vi "Camera_init.vi"(8 "error in":errorcluster, 11 "input cluster":T1={"L16 Linear Actuator"="", "XE 1000 Pump"="", "Camera1"="", "Camera2"="", "Img_Capt"=FALSE, "Actuator"=FALSE, "Pump"=FALSE, "Cam 1"=FALSE, "Cam 2"=FALSE, "Empty_Refill"=FALSE, "Crop"=FALSE, "Light intensity"=100, "Exposure Time"=1000.0, "Sample Name"="Test Sample", "Operator"="MRJ", "Calibration 1"=path "C:/Users/au540322/Desktop/IHS_Project/images/Debris/Debris_0/Debris_0_2019_06_01-23-32-49-686.PNG", "Calibration 2"=path "C:/Users/au540322/Desktop/IHS_Project/images/Debris/Debris_0/Debris_0_2019_06_01-23-32-49-686.PNG", "Framerate"=1, "Timeout Sample"=0, "Collection date"="MRJ", "Sample size threshold"=1, "Empty start"=1, "Command"="MRJ", "Station"="", "Species Name"="", "Other Notes"="", "Aperture"=enum."Item 0", "Image Process Queue Size"=500, "Image Save Queue Size"=500, "Overload threshold"=500, "Max Framerate"=100, "Rectangle 1"={"Left"=0, "Top"=0, "Right"=0, "Bottom"=0, "Rotation"=0.0}, "Rectangle 2"={"Left"=0, "Top"=0, "Right"=0, "Bottom"=0, "Rotation"=0.0}, "Detection Region %"=0.0, "Detect 1"=path "C:/Users/au540322/Desktop/IHS_Project/images/Debris/Debris_0/Debris_0_2019_06_01-23-32-49-686.PNG", "Detect 2"=path "C:/Users/au540322/Desktop/IHS_Project/images/Debris/Debris_0/Debris_0_2019_06_01-23-32-49-686.PNG", "Max large object threshold"=0, "Open(T)/Close(F)"=FALSE, "Img_Capt Begin"=FALSE, "Dispense Speed"=100, "Flush Size"=100, "Location"="Station", "Latitude"="Station", "Longitude"="Station", "Determiner"="Station", "Sex"="Station", "Camera1_Img"=refnum, "Camera2_Img"=refnum, "Img1_Orig_Disp"=refnum, "Img2_Orig_Disp"=refnum, "Img1_Orig_RGB"=refnum, "Img2_Orig_RGB"=refnum, "Blue_Plane_Extract"=refnum, "Subtracted_Plane"=refnum, "Img1_Binary"=refnum, "Img2_Binary"=refnum, "Crop_Mask"=refnum, "Img1_Save"=refnum, "Img2_Save"=refnum, "Img1_Cali_Full"=refnum, "Img2_Cali_Full"=refnum, "Img1_Cali_Detect"=refnum, "Img2_Cali_Detect"=refnum, "Cam 1 queue"=refnum, "Cam 2 queue"=refnum, "Cam 1 - save queue"=refnum, "Cam 2 - save queue"=refnum, "Overlay_Ring"=0, "SystemVersion"=0, "System Serial"="", "Legacy Cam Attributes"=FALSE, "Camera Orientation 1"="", "Camera Orientation 2"="", "Pixel to mm 1"=0.0, "Pixel to mm 2"=0.0} {"SystemVersion" items=["Standard", "XL"]; "Overlay_Ring" items=["Session Data", "Extended Setup", "Buffer", "Camera", "Dispenser", "Stats", "Connections"]; "Flush Size" min=1; "Dispense Speed" min=1; "Rectangle 2"."Rotation" format="%.2f"; "Rectangle 2"."Left" scale=0.0..1024.0; "Rectangle 2"."Right" scale=0.0..1024.0; "Rectangle 1"."Rotation" format="%.2f"; "Rectangle 1"."Left" scale=0.0..1024.0; "Rectangle 1"."Right" scale=0.0..1024.0; "Max Framerate" min=1; "Overload threshold" min=1; "Image Save Queue Size" min=1; "Image Process Queue Size" min=1; "Empty start" min=1; "Sample size threshold" min=1; "Framerate" min=1; "Light intensity" scale=0.0..100.0}) -> (0 "Cam2 Status":bool, 1 "Cam1 Status":bool, 2 "Camera2":T2, 3 "Camera1":T2)   [LabVIEW 2022 SP3]
uses:
  <vilib>/userdefined/High Color/IMAQdx.ctl
  controls/Data.ctl
  <vilib>/vision/Image Controls.llb/IMAQ Image.ctl
  <vilib>/vision/driver/IMAQdx.llb/IMAQdx Camera Control Mode.ctl
  5e997588-f8a4-47c3-81e2-b2b6234dc64e.vi
  <vilib>/vision/driver/NI_Vision_Acquisition_Software.lvlib
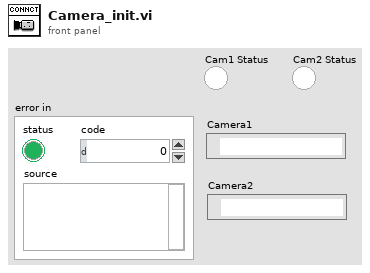
[diagram p1: front panel]
types:
  T1 = typedef "Data.ctl" = cluster{"L16 Linear Actuator":refnum<visa-resource-name>, "XE 1000 Pump":refnum<visa-resource-name>, "Camera1":T2, "Camera2":T2, "Img_Capt":bool, "Actuator":bool, "Pump":bool, "Cam 1":bool, "Cam 2":bool, "Empty_Refill":bool, "Crop":bool, "Light intensity":i32, "Exposure Time":dbl, "Sample Name":string, "Operator":string, "Calibration 1":path, "Calibration 2":path, "Framerate":i32, "Timeout Sample":i32, "Collection date":string, "Sample size threshold":i32, "Empty start":u32, "Command":string, "Station":string, "Species Name":string, "Other Notes":string, "Aperture":enum32{"Item 0", "Item 1", "Item 2", "Item 3"}, "Image Process Queue Size":i32, "Image Save Queue Size":i32, "Overload threshold":i32, "Max Framerate":i32, "Rectangle 1":T3, "Rectangle 2":T3, "Detection Region %":dbl, "Detect 1":path, "Detect 2":path, "Max large object threshold":i32, "Open(T)/Close(F)":bool, "Img_Capt Begin":bool, "Dispense Speed":i32, "Flush Size":i32, "Location":string, "Latitude":string, "Longitude":string, "Determiner":string, "Sex":string, "Camera1_Img":T4, "Camera2_Img":T4, "Img1_Orig_Disp":T4, "Img2_Orig_Disp":T4, "Img1_Orig_RGB":T4, "Img2_Orig_RGB":T4, "Blue_Plane_Extract":T4, "Subtracted_Plane":T4, "Img1_Binary":T4, "Img2_Binary":T4, "Crop_Mask":T4, "Img1_Save":T4, "Img2_Save":T4, "Img1_Cali_Full":T4, "Img2_Cali_Full":T4, "Img1_Cali_Detect":T4, "Img2_Cali_Detect":T4, "Cam 1 queue":refnum<queue>, "Cam 2 queue":refnum<queue>, "Cam 1 - save queue":refnum<queue>, "Cam 2 - save queue":refnum<queue>, "Overlay_Ring":u16, "SystemVersion":u16, "System Serial":string, "Legacy Cam Attributes":bool, "Camera Orientation 1":string, "Camera Orientation 2":string, "Pixel to mm 1":dbl, "Pixel to mm 2":dbl}
  T2 = typedef "IMAQdx.ctl" = refnum<k21>
  T3 = typedef "IMAQ Rectangle" = cluster{"Left":i32, "Top":i32, "Right":i32, "Bottom":i32, "Rotation":dbl}
  T4 = typedef "IMAQ Image.ctl" = refnum<image>
  T5 = typedef "CAM_ID.ctl" = cluster{"CAM_ID1":i32, "CAM_ID2":i32}
  T6 = typedef "NI_Vision_Acquisition_Software.lvlib/IMAQdx Camera Control Mode.ctl" = enum32{"Controller", "Listener"}
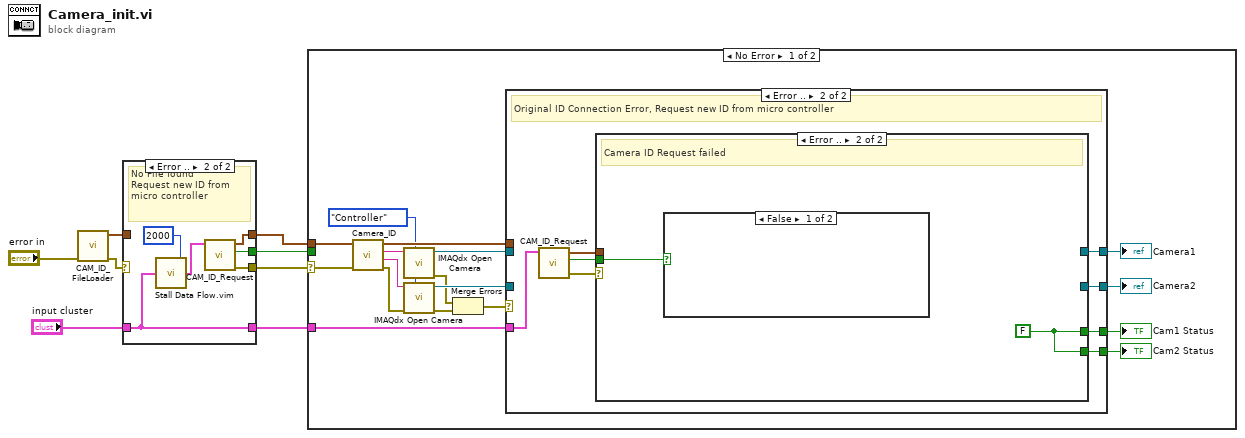
[diagram p0: block diagram]
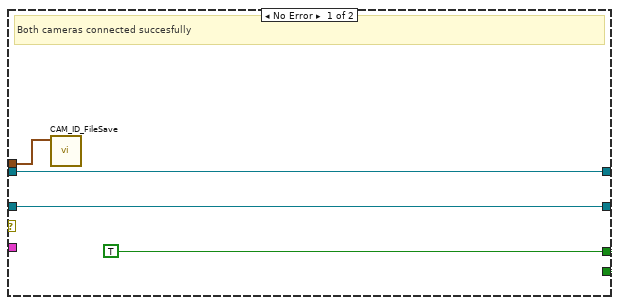
[diagram p2: hidden frame]
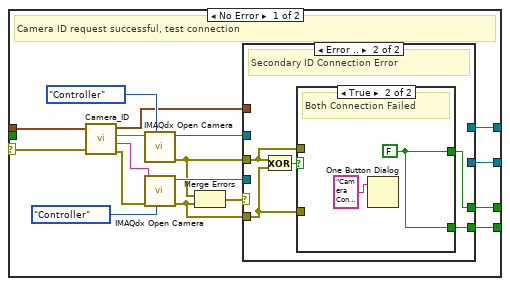
[diagram p3: hidden frame]
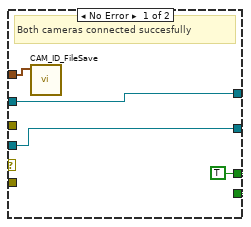
[diagram p4: hidden frame]
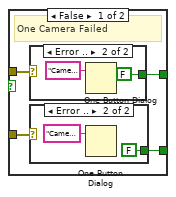
[diagram p5: hidden frame]
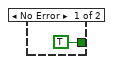
[diagram p6: hidden frame]
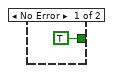
[diagram p7: hidden frame]
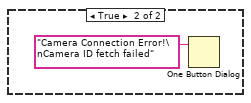
[diagram p8: hidden frame]
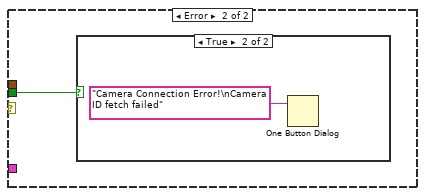
[diagram p9: hidden frame]
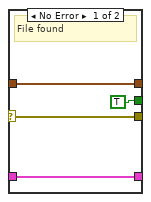
[diagram p11: hidden frame]
diagram:
  n1 = call "CAM_ID_FileLoader.vi"("error in"="error in") -> ("error out"=w6:errorcluster, "CAM_ID"=w8:T5)  [unwired: 9 in]
  n2 = case shown="Error .." w6 {
    selector: w6 -> [w11 _]
    tunnel: [w12 w18] -> w7
    tunnel: w8 -> [w12 _]
    tunnel: "input cluster" -> [w10 w14]
    tunnel: [w11 w17] -> w4
    tunnel: [w10 w14] -> w2
    tunnel: [TRUE ("Connection?") w13] -> w1
    frame No Error {
      # "File found"
    }
    frame Error {
      # "No File found\nRequest new ID from micro controller"
      n3 = call "Stall Data Flow.vim"("value in"=w14, "milliseconds to wait"=u32 2000) -> ("value out"=w15:T1)  [unwired: 1 out]
      n4 = call "CAM_ID_Request.vi"("input cluster"=w15) -> ("error out"=w17:errorcluster, "Connection?"=w13:bool, "CAM_ID"=w18:T5)  [unwired: 8 in]
    }
  }
  n5 = case shown="No Error" w4 {
    selector: w4 -> [w31 _]
    tunnel: w7 -> [w34 _]
    tunnel: w2 -> [w24 _]
    tunnel: w1 -> [_ w89]
    frame No Error {
      w21 = IMAQdx_Camera_Control_Mode."Controller" ("Camera Control Mode")
      n6 = call "Camera_ID.vi"("error in"=w31, "CAM_ID"=w34) -> ("error out"=w35:errorcluster, "CAM2"=w33:string, "CAM1"=w26:string, "CAM_ID out"=w27:T5)  [unwired: 6 in]
      n7 = call <vilib>:"IMAQdx Open Camera.vi"("Camera Control Mode"=w21, "Session In"=w26) -> ("error out"=w30:errorcluster, "Session Out"=w25:T2)  [unwired: 8 in]
      n8 = call <vilib>:"IMAQdx Open Camera.vi"("Camera Control Mode"=w21, "error in"=w35, "Session In"=w33) -> ("error out"=w29:errorcluster, "Session Out"=w32:T2)  [unwired: 7 in]
      n9 = Merge Errors(w30, w29) -> (w28:errorcluster)
      n10 = case shown="Error .." w28 {
        tunnel: w32 -> [w37 _]
        tunnel: w27 -> [w39 _]
        tunnel: w25 -> [w38 _]
        tunnel: w24 -> [_ w47]
        tunnel: [w38 w45] -> w23
        tunnel: [w37 w44] -> w22
        tunnel: [w36 w43] -> w20
        tunnel: [w36 w42] -> w19
        frame No Error {
          w36 = TRUE
          # "Both cameras connected succesfully"
          n11 = call "CAM_ID_FileSave.vi"("CAM_ID"=w39) -> ()  [unwired: 11 in]
        }
        frame Error {
          # "Original ID Connection Error, Request new ID from micro controller"
          n12 = call "CAM_ID_Request.vi"("input cluster"=w47) -> ("error out"=w41:errorcluster, "Connection?"=w40:bool, "CAM_ID"=w46:T5)  [unwired: 8 in]
          n13 = case shown="Error .." w41 {
            selector: w41 -> [w48 _]
            tunnel: w46 -> [w59 _]
            tunnel: [w54 _] -> w45
            tunnel: [w53 _] -> w44
            tunnel: [w50 w87] -> w43
            tunnel: [w49 w87] -> w42
            tunnel: w40 -> [_ w86]
            frame No Error {
              # "Camera ID request successful, test connection"
              n14 = call "Camera_ID.vi"("error in"=w48, "CAM_ID"=w59) -> ("error out"=w60:errorcluster, "CAM2"=w63:string, "CAM1"=w64:string, "CAM_ID out"=w55:T5)  [unwired: 6 in]
              n15 = call <vilib>:"IMAQdx Open Camera.vi"("Camera Control Mode"=IMAQdx_Camera_Control_Mode."Controller", "Session In"=w64) -> ("error out"=w52:errorcluster, "Session Out"=w56:T2)  [unwired: 8 in]
              n16 = call <vilib>:"IMAQdx Open Camera.vi"("Camera Control Mode"=IMAQdx_Camera_Control_Mode."Controller", "error in"=w60, "Session In"=w63) -> ("error out"=w51:errorcluster, "Session Out"=w57:T2)  [unwired: 7 in]
              n17 = Merge Errors(w52, w51) -> (w58:errorcluster)
              n18 = case shown="Error .." w58 {
                tunnel: w57 -> [w66 _]
                tunnel: w56 -> [w67 _]
                tunnel: w55 -> [w68 _]
                tunnel: [w67 _] -> w54
                tunnel: [w66 _] -> w53
                tunnel: w52 -> [_ w72]
                tunnel: w51 -> [_ w71]
                tunnel: [w65 w69] -> w50
                tunnel: [w65 w70] -> w49
                frame No Error {
                  w65 = TRUE
                  # "Both cameras connected succesfully"
                  n19 = call "CAM_ID_FileSave.vi"("CAM_ID"=w68) -> ()  [unwired: 11 in]
                }
                frame Error {
                  # "Secondary ID Connection Error"
                  n20 = Exclusive Or(1:w71, 2:w72) -> (0:w73:bool)
                  n21 = case shown="True" w73 {
                    tunnel: w72 -> [w77 _]
                    tunnel: w71 -> [w76 _]
                    tunnel: [w75 w85] -> w70
                    tunnel: [w74 w85] -> w69
                    frame False {
                      # "One Camera Failed"
                      n22 = case shown="Error .." w77 {
                        tunnel: [TRUE FALSE] -> w75
                        frame No Error {
                        }
                        frame Error {
                          n23 = One Button Dialog(message="Camera 1 connection error") -> ()  [unwired: 1 in, 1 out]
                        }
                      }
                      n24 = case shown="Error .." w76 {
                        tunnel: [TRUE FALSE] -> w74
                        frame No Error {
                        }
                        frame Error {
                          n25 = One Button Dialog(message="Camera 2 connection error") -> ()  [unwired: 1 in, 1 out]
                        }
                      }
                    }
                    frame True {
                      w85 = FALSE
                      # "Both Connection Failed"
                      n26 = One Button Dialog(message="Camera Connection Error!\nCamera Connect Failed") -> ()  [unwired: 1 in, 1 out]
                    }
                  }
                }
              }
            }
            frame Error {
              w87 = FALSE
              # "Camera ID Request failed"
              n27 = case shown="False" w86 {
                frame False {
                }
                frame True {
                  n28 = One Button Dialog(message="Camera Connection Error!\nCamera ID fetch failed") -> ()  [unwired: 1 in, 1 out]
                }
              }
            }
          }
        }
      }
      "Camera1" <- w23
      "Camera2" <- w22
      "Cam1 Status" <- w19
      "Cam2 Status" <- w20
    }
    frame Error {
      n29 = case shown="True" w89 {
        frame False {
        }
        frame True {
          n30 = One Button Dialog(message="Camera Connection Error!\nCamera ID fetch failed") -> ()  [unwired: 1 in, 1 out]
        }
      }
    }
  }
